vi "Get Expected Brightness.vi"(7 "I_Mixed Coordinates":i32[][](array[numeric]), 8 "I_Sigma":i16, 9 "I_Number of columns":i16, 10 "I_Number of rows":i16, 11 "I_Blue Component":u8[](array[numeric])) -> (3 "O_Text":i16[](array[numeric]))   [LabVIEW 2015]
panel:
  out "Array 2":dbl[](array[numeric])
  out "Array":u8[](array[numeric])
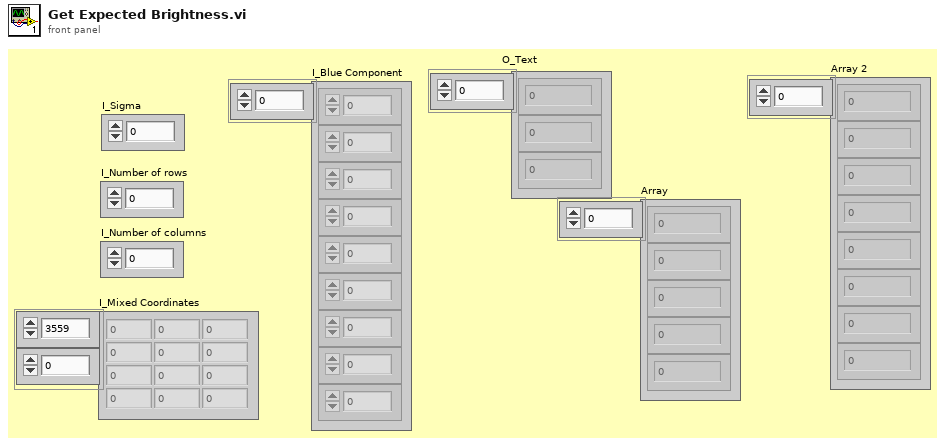
[diagram p1: front panel]
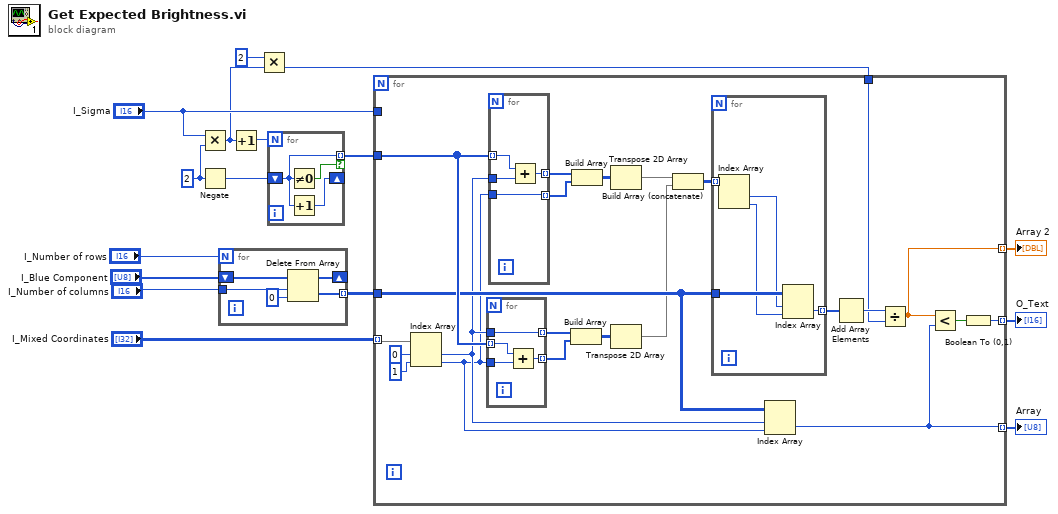
[diagram p0: block diagram]
diagram:
  w11 = i16 2 ("y")
  n1 = Multiply(x="I_Sigma", y=w11) -> (x*y=w6:i16)
  n2 = Negate(x=w11) -> (-x=w10:i16)
  n3 = for {
    N: "I_Number of rows" -> [_]
    tunnel: "I_Number of columns" -> [w20]
    shift-right: [w18] -> _
    shift-left: "I_Blue Component" -> [w21]
    tunnel: [w17] -> w13 mode=indexing
    n4 = Delete From Array(array=w21, length=w20, index=0) -> (deleted portion=w17:u8[], array with subset deleted=w18:u8[])
  }
  n5 = Increment(x=w6) -> (x+1=w9:i16)
  n6 = Multiply(x=i16 2, y=w6) -> (x*y=w4:i16)
  n7 = for {
    N: w9 -> [_]
    shift-right: [w24] -> _
    shift-left: w10 -> [w23]
    tunnel: [w23] -> w7 mode=indexing if=w22
    n8 = Not Equal To 0?(x=w23) -> (x != 0?=w22:bool)
    n9 = Increment(x=w23) -> (x+1=w24:i16)
  }
  n10 = for {
    tunnel: w13 -> [w37]
    tunnel: "I_Sigma" -> [_]
    tunnel: "I_Mixed Coordinates" -> [w47] mode=indexing
    tunnel: w7 -> [w46]
    tunnel: w4 -> [w33]
    tunnel: [w31] -> w5 mode=indexing
    tunnel: [w30] -> w2 mode=indexing
    tunnel: [w27] -> w1 mode=indexing
    n11 = Index Array(array=w47, index #1=0 ("index"), index #2=1 ("index")) -> (element #1=w36:i32, element #2=w35:i32)
    n12 = for {
      tunnel: w46 -> [w55] mode=indexing
      tunnel: w35 -> [w56]
      tunnel: [w54] -> w43 mode=indexing
      tunnel: w36 -> [w54]
      tunnel: [w53] -> w42 mode=indexing
      n13 = Add(x=w55, y=w56) -> (x+y=w53:i32)
    }
    n14 = for {
      tunnel: w46 -> [w59] mode=indexing
      tunnel: w36 -> [w60]
      tunnel: w35 -> [w57]
      tunnel: [w58] -> w45 mode=indexing
      tunnel: [w57] -> w44 mode=indexing
      n15 = Add(x=w59, y=w60) -> (x+y=w58:i32)
    }
    n16 = Build Array(w43, w42) -> (w40:i32[][])
    n17 = Build Array(w45, w44) -> (w41:i32[][])
    n18 = Transpose 2D Array(2D array=w41) -> (transposed array=w26:i32[][])
    n19 = Transpose 2D Array(2D array=w40) -> (transposed array=w25:i32[][])
    n20 = Build Array (concatenate)(w26, w25) -> (w39:i32[][])
    n21 = for {
      tunnel: w39 -> [w52] mode=indexing
      tunnel: w37 -> [w51]
      tunnel: [w48] -> w38 mode=indexing
      n22 = Index Array(array=w52) -> (element #1=w50:i32, element #2=w49:i32)  [unwired: 2 in]
      n23 = Index Array(array=w51, index (row)=w50, index (col)=w49) -> (element=w48:u8)
    }
    n24 = Index Array(array=w37, index (row)=w36, index (col)=w35) -> (element=w30:u8)
    n25 = Add Array Elements(numeric array=w38) -> (sum=w34:u8)
    n26 = Divide(x=w34, y=w33) -> (x/y=w27:dbl)
    n27 = Less?(x=w27, y=w30) -> (x < y?=w32:bool)
    n28 = Boolean To (0,1)(Boolean=w32) -> (0, 1=w31:i16)
  }
  "O_Text" <- w5
  "Array" <- w2
  "Array 2" <- w1
